vi "ASIC_READ.vi"(7 "Espera acceso USB":u32, 8 "error in":errorcluster, 10 "Direccion Registro Asic":u8 format="%x", 11 "ftHandle_in":u32) -> (0 "error out":errorcluster, 2 "Valor Asic":u16 format="%x", 3 "ftHandle_out":u32)   [LabVIEW 2019]
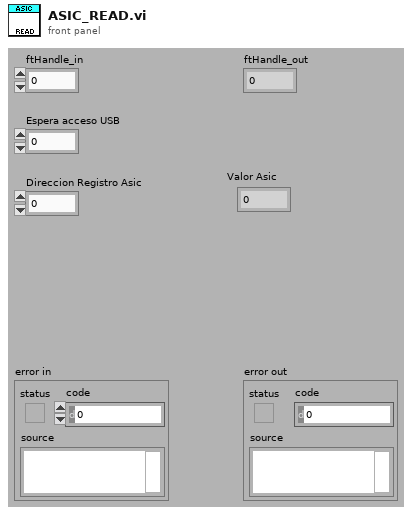
[diagram p1: front panel]
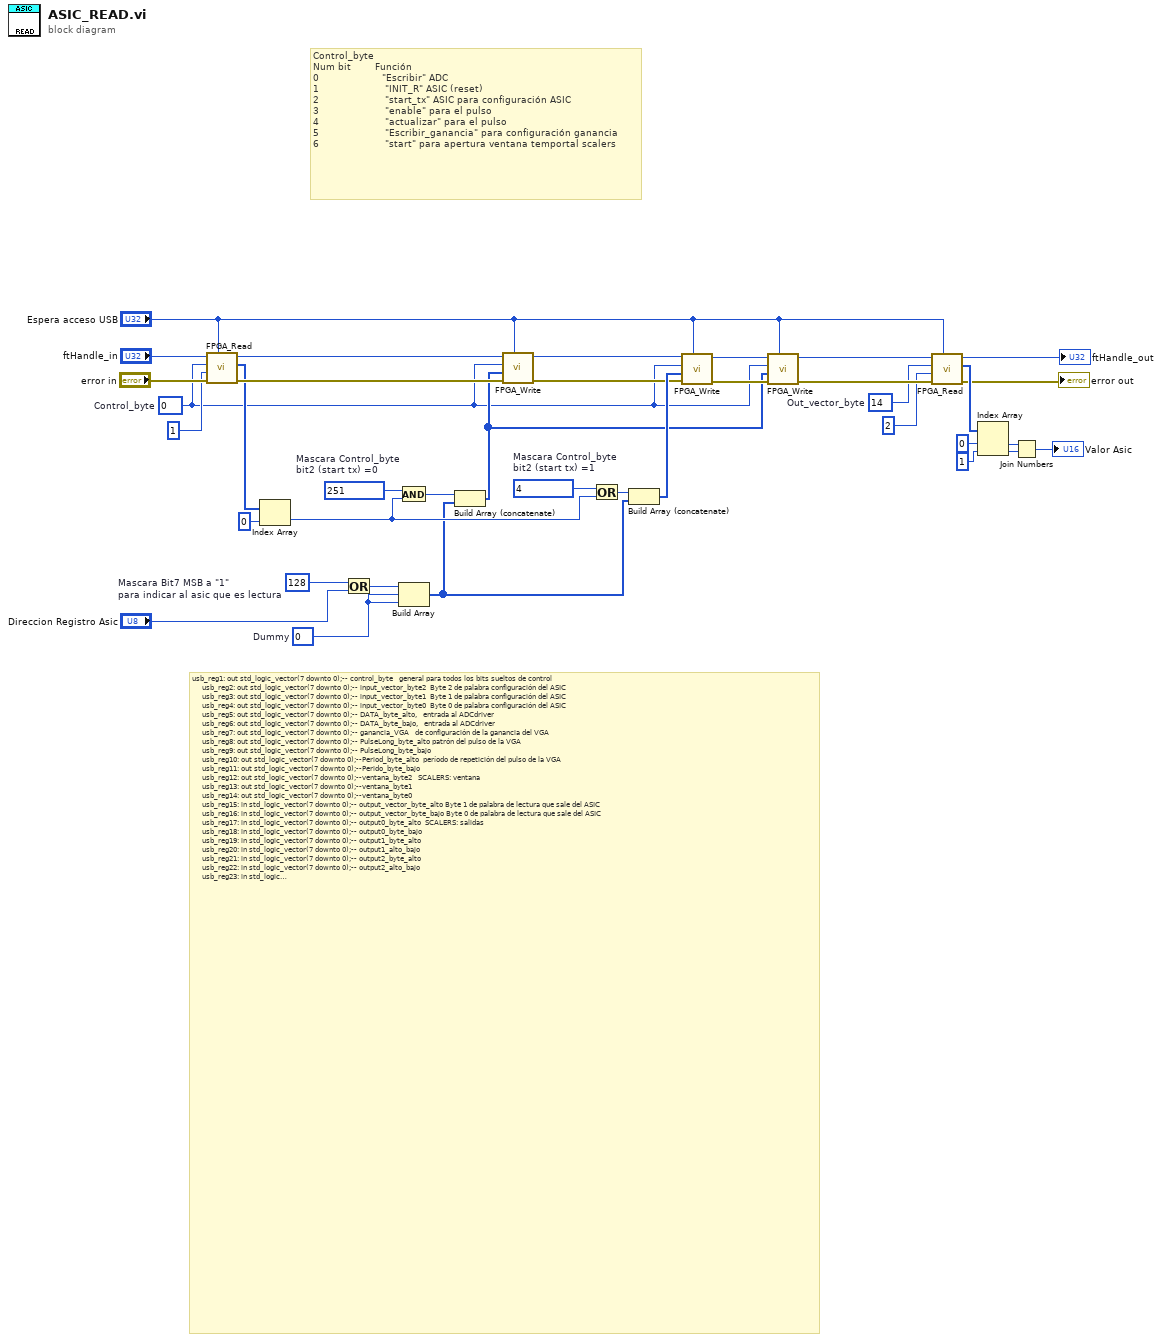
[diagram p0: block diagram]
diagram:
  w1 = u8 0  # Dummy
  w12 = u8 14  # Out_vector_byte
  w23 = u8 4  # Mascara Control_byte bit2 (start tx) =1
  w35 = u8 128  # Mascara Bit7 MSB a "1" para indicar al asic que es lectura
  w15 = u8 0  # Control_byte
  w28 = u8 251  # Mascara Control_byte bit2 (start tx) =0
  # "usb_reg1: out std_logic_vector(7 downto 0);-- control_byte\t\t\tgeneral para todos los bits sueltos de control\n\t\t\t  usb_reg2: out std_logic_vector(7 downto 0);-- input_vector_byte2 \tByte 2 de palabra configuración del ASIC\n\t\t\t  usb_reg3: out std_logic_vector(7 downto 0);-- input_vector_byte1 \tByte 1 de palabra configuración del ASIC\n\t\t\t  usb_reg4: out std_logic_vector(7 downto 0);-- input_vector_byte0 \tByte 0 de palabra configuración del ASIC\n\t\t\t  usb_reg5: out std_logic_vector(7 downto 0);-- DATA_byte_alto, \t\tentrada al ADCdriver\n\t\t\t  usb_reg6: out std_logic_vector(7 downto 0);-- DATA_byte_bajo, \t\tentrada al ADCdriver\n\t\t\t  usb_reg7: out std_logic_vector(7 downto 0);-- ganancia_VGA\t\t\tde configuración de la ganancia del VGA\n\t\t\t  usb_reg8: out std_logic_vector(7 downto 0);-- PulseLong_byte_alto\tpatrón del pulso de la VGA\n\t\t\t  usb_reg9: out std_logic_vector(7 downto 0);-- PulseLong_byte_bajo\n\t\t\t  usb_reg10: out std_logic_vector(7 downto 0);--Period_byte_alto\t\tperíodo de repetición del pulso de la VGA\n\t\t\t  usb_reg11: out std_logic_vector(7 downto 0);--Perido_byte_bajo\n\t\t\t  usb_reg12: out std_logic_vector(7 downto 0);--ventana_byte2\t\t\tSCALERS: ventana\n\t\t\t  usb_reg13: out std_logic_vector(7 downto 0);--ventana_byte1\t\n\t\t\t  usb_reg14: out std_logic_vector(7 downto 0);--ventana_byte0\n\t\t\t  usb_reg15: in std_logic_vector(7 downto 0);-- output_vector_byte_alto\tByte 1 de palabra de lectura que sale del ASIC\n\t\t\t  usb_reg16: in std_logic_vector(7 downto 0);-- output_vector_byte_bajo\tByte 0 de palabra de lectura que sale del ASIC\n\t\t\t  usb_reg17: in std_logic_vector(7 downto 0);-- output0_byte_alto\t\tSCALERS: salidas\n\t\t\t  usb_reg18: in std_logic_vector(7 downto 0);-- output0_byte_bajo\n\t\t\t  usb_reg19: in std_logic_vector(7 downto 0);-- output1_byte_alto\n\t\t\t  usb_reg20: in std_logic_vector(7 downto 0);-- output1_alto_bajo \n\t\t\t  usb_reg21: in std_logic_vector(7 downto 0);-- output2_byte_alto \n\t\t\t  usb_reg22: in std_logic_vector(7 downto 0);-- output2_alto_bajo \n\t\t\t  usb_reg23: in std_logic_vector(7 downto 0);-- para el canal_0 del ADCdriver\n\t\t\t  usb_reg24: in std_logic_vector(7 downto 0);\n\t\t\t  usb_reg25: in std_logic_vector(7 downto 0);-- para el canal_1 del ADCdriver\n\t\t\t  usb_reg26: in std_logic_vector(7 downto 0);\n\t\t\t  usb_reg27: in std_logic_vector(7 downto 0);-- para el canal_2 del ADCdriver\n\t\t\t  usb_reg28: in std_logic_vector(7 downto 0);\n\t\t\t  usb_reg29: in std_logic_vector(7 downto 0);-- para el canal_3 del ADCdriver\n\t\t\t  usb_reg30: in std_logic_vector(7 downto 0);\n\t\t\t  usb_reg31: in std_logic_vector(7 downto 0);-- para el canal_4 del ADCdriver\n\t\t\t  usb_reg32: in std_logic_vector(7 downto 0);\n\t\t\t  usb_reg33: in std_logic_vector(7 downto 0);-- para el canal_5 del ADCdriver\n\t\t\t  usb_reg34: in std_logic_vector(7 downto 0);\n\t\t\t  usb_reg35: in std_logic_vector(7 downto 0);-- para el canal_6 del ADCdriver\n\t\t\t  usb_reg36: in std_logic_vector(7 downto 0);\n\t\t\t  usb_reg37: in std_logic_vector(7 downto 0);-- para el canal_7 del ADCdriver\n\t\t\t  usb_reg38: in std_logic_vector(7 downto 0);\n\t\t\t  usb_reg39: in std_logic_vector(7 downto 0);-- para el canal_8 del ADCdriver\n\t\t\t  usb_reg40: in std_logic_vector(7 downto 0);\n\t\t\t  usb_reg41: in std_logic_vector(7 downto 0);-- para el canal_9 del ADCdriver\n\t\t\t  usb_reg42: in std_logic_vector(7 downto 0);\n\t\t\t  usb_reg43: in std_logic_vector(7 downto 0);-- para el canal_10 del ADCdriver\n\t\t\t  usb_reg44: in std_logic_vector(7 downto 0)--;"
  # "Control_byte\nNum bit        Función\n0                     \"Escribir\" ADC\n1                      \"INIT_R\" ASIC (reset)\n2                      \"start_tx\" ASIC para configuración ASIC\n3                      \"enable\" para el pulso\n4                      \"actualizar\" para el pulso\n5                      \"Escribir_ganancia\" para configuración ganancia\n6                      \"start\" para apertura ventana temportal scalers"
  n1 = call "FPGA_Read.vi"("Espera acceso USB"="Espera acceso USB", "error in"="error in", "Numero Bytes"=u8 1, "Dirección base"=w15, "ftHandle_in"="ftHandle_in") -> ("error out"=w32:errorcluster, "lpBuffer_out"=w30:u8[])  [unwired: 2 in, 3 out]
  n2 = Index Array(array=w30, index=0) -> (element=w24:u8)
  n3 = Or(x=w35, y="Direccion Registro Asic") -> (x .or. y?=w26:u8)
  n4 = And(x=w28, y=w24) -> (x .and. y?=w25:u8)
  n5 = Build Array ("Escribimos en usb reg1, reg2, reg3 y reg4")(w26, w1, w1) -> (w19:u8[])
  n6 = Build Array (concatenate) ("Escribimos en usb reg1, reg2, reg3 y reg4")(w25, w19) -> (w16:u8[])
  n7 = call "FPGA_Write.vi"("Espera acceso USB"="Espera acceso USB", "error in"=w32, "Bytes de escritura"=w16, "Dirección base"=w15, "ftHandle_in"="ftHandle_in") -> ("error out"=w20:errorcluster, "ftHandle_out"=w27:u32)  [unwired: 1 in, 2 out]
  n8 = Or(x=w23, y=w24) -> (x .or. y?=w22:u8)
  n9 = Build Array (concatenate) ("Escribimos en usb reg1, reg2, reg3 y reg4")(w22, w19) -> (w21:u8[])
  n10 = call "FPGA_Write.vi"("Espera acceso USB"="Espera acceso USB", "error in"=w20, "Bytes de escritura"=w21, "Dirección base"=w15, "ftHandle_in"=w27) -> ("error out"=w17:errorcluster, "ftHandle_out"=w18:u32)  [unwired: 1 in, 2 out]
  n11 = call "FPGA_Write.vi"("Espera acceso USB"="Espera acceso USB", "error in"=w17, "Bytes de escritura"=w16, "Dirección base"=w15, "ftHandle_in"=w18) -> ("error out"=w13:errorcluster, "ftHandle_out"=w14:u32)  [unwired: 1 in, 2 out]
  n12 = call "FPGA_Read.vi"("Espera acceso USB"="Espera acceso USB", "error in"=w13, "Numero Bytes"=u8 2, "Dirección base"=w12, "ftHandle_in"=w14) -> ("error out"=→"error out":errorcluster, "lpBuffer_out"=w10:u8[], "ftHandle_out"=→"ftHandle_out":u32)  [unwired: 2 in, 2 out]
  n13 = Index Array(array=w10, index #1=0 ("index"), index #2=1 ("index")) -> (element #1=w6:u8, element #2=w7:u8)
  n14 = Join Numbers(hi=w6, lo=w7) -> ((hi.lo)=→"Valor Asic":u16)
